vi "Global Cancel Control.vi"() -> ()   [LabVIEW 2020]
uses:
  Globals and TypeDefs/Global Varibal Control.vi
panel:
  in  "Resume":bool
  in  "Cancel":bool
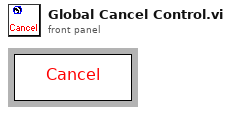
[diagram p1: front panel]
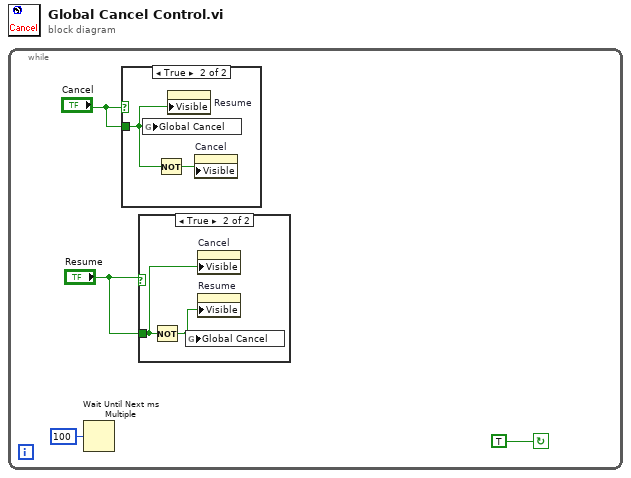
[diagram p0: block diagram]
diagram:
  n1 = while {
    stop <- TRUE continue-if-true
    n2 = Wait Until Next ms Multiple(millisecond multiple=u32 100) -> ()  [unwired: 1 out]
    n3 = case shown="True" "Cancel" {
      tunnel: "Cancel" -> [_ w7]
      frame False {
      }
      frame True {
        n4 = global write "Global Varibal Control.vi" "Global Cancel"(w7) -> ()
        n5 = Not(x=w7) -> (.not. x?=w8:bool)
        n6 = property on="Resume" class="Bool"("Visible"=w7) -> ()  [unwired: 2 in, 2 out]
        n7 = property on="Cancel" class="Bool"("Visible"=w8) -> ()  [unwired: 2 in, 2 out]
      }
    }
    n8 = case shown="True" "Resume" {
      tunnel: "Resume" -> [_ w6]
      frame False {
      }
      frame True {
        n9 = Not(x=w6) -> (.not. x?=w5:bool)
        n10 = global write "Global Varibal Control.vi" "Global Cancel"(w5) -> ()
        n11 = property on="Cancel" class="Bool"("Visible"=w6) -> ()  [unwired: 2 in, 2 out]
        n12 = property on="Resume" class="Bool"("Visible"=w5) -> ()  [unwired: 2 in, 2 out]
      }
    }
  }
